vi "Update Position Status.vi"(11 "Movable in":refnum<class "Movable.lvclass">) -> (3 "Movable out":refnum<class "Movable.lvclass">)   [LabVIEW 2024, in "Movable.lvclass"]
doc: "MIT Licence\nCopyright (c) 2024 David Grollier"
uses:
  Movable.lvclass
  Movable.lvclass/Movable.ctl
  Game Componants.lvclass/Game Componants.ctl
  Game Componants.lvclass
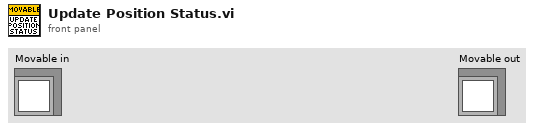
[diagram p1: front panel]
types:
  T1 = typedef "Coordinates.ctl" = cluster{"x":dbl, "y":dbl}
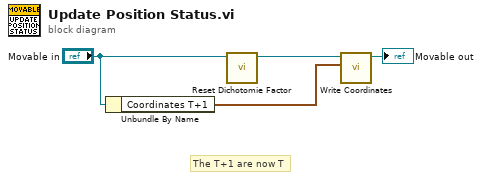
[diagram p0: block diagram]
diagram:
  # "The T+1 are now T"
  n1 = Unbundle By Name("Movable in") -> ("Coordinates T+1"=w3:T1)
  n2 = call "Reset Dichotomie Factor.vi"("Movable in"="Movable in") -> ("Movable out"=w4:refnum<class "Movable.lvclass">)  [unwired: 10 in]
  n3 = call "Write Coordinates.vi"("Coordinates"=w3, "Game Componants in"=w4) -> ("Game Componants out"=→"Movable out":refnum<class "Movable.lvclass">)  [unwired: 9 in]
